vi "PCO_GetPendingBuffer.vi"(8 "error in (no error)":errorcluster, 11 "Handle":u64) -> (0 "error out":errorcluster, 2 "icount":i32, 3 "Handle Out":u64, 5 "return type":u32 format="%x")   [LabVIEW 2011]
uses:
  SC2_Cam64.dll
panel:
  # "Arms, i.e. prepares the camera for a consecutive set recording status = [run] command. All \nconfigurations and settings made up to this moment are accepted and the internal settings of the \ncamera are prepared. Thus the camera is able to start immediately when the set recording status \n= [run] command is performed.\nNote:  It is required to issue an arm camera command before every set recording state = [run] \ncommand in order to ensure that all settings are accepted correctly. Do not change settings \nbetween arm camera command and set recording status command."
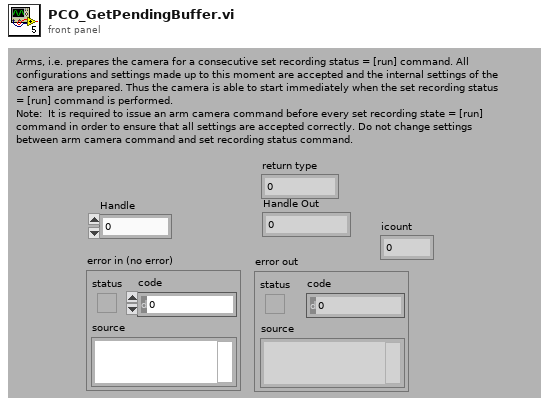
[diagram p1: front panel]
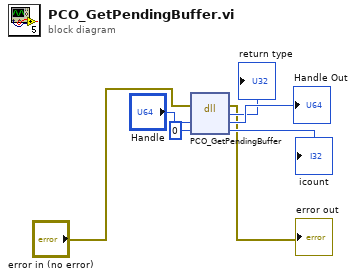
[diagram p0: block diagram]
diagram:
  n1 = dll-call lib="SC2_Cam*.*" fn="PCO_GetPendingBuffer"(error in="error in (no error)", "Handle"="Handle", "icount"=0) -> (error out=→"error out":errorcluster, "return type"=→"return type":u32, "Handle"=→"Handle Out":u64, "icount"=→"icount":i32)  [unwired: 2 in, 1 out]
